vi "Timeout action.vi"(8 "error in (no error)":errorcluster, 11 "Loop data in":T1={"Config"={"List"=[], "max rows"=8, "Listbox placement"=enum."None", "String Color Options"={"Use? (F)"=FALSE, "Color - Valid"=0, "Color - Invalid"=0, "Allow blank?"=FALSE}}, "Refs"={"String"=refnum, "Listbox"=refnum}, "State"={"LB active?"=FALSE}}) -> (0 "error out":errorcluster, 3 "Loop data out":T1={"Config"={"List"=[], "max rows"=8, "Listbox placement"=enum."None", "String Color Options"={"Use? (F)"=FALSE, "Color - Valid"=0, "Color - Invalid"=0, "Allow blank?"=FALSE}}, "Refs"={"String"=refnum, "Listbox"=refnum}, "State"={"LB active?"=FALSE}})   [LabVIEW 2021, in "Autocomplete Textbox.lvlib"]
uses:
  Autocomplete Textbox.lvlib
  Loop Data.ctl
  Inputs.ctl
  Classes/Handle/Listbox placement.ctl
  Color String Options.ctl
  Refs.ctl
  State data.ctl
  Classes/Handle/Handle.lvclass
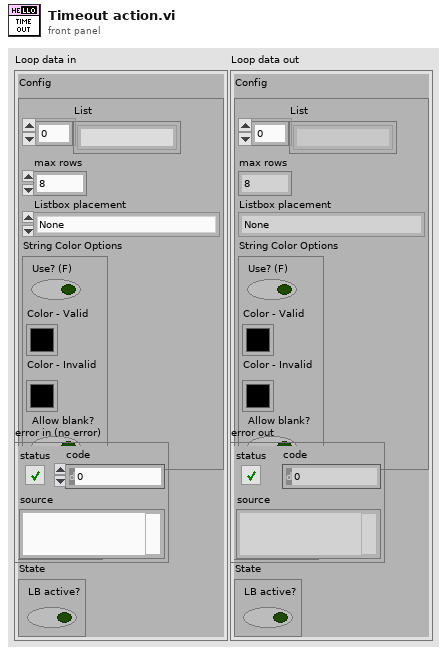
[diagram p1: front panel]
types:
  T1 = typedef "Autocomplete Textbox.lvlib/Loop Data.ctl" = cluster{"Config":T2, "Refs":T5, "State":T6}
  T2 = typedef "Autocomplete Textbox.lvlib/Inputs.ctl" = cluster{"List":string[], "max rows":i32, "Listbox placement":T3, "String Color Options":T4}
  T3 = typedef "Autocomplete Textbox.lvlib/Handle.lvclass/Listbox placement.ctl" = enum16{"None", "Under String", "Fit to Pane"}
  T4 = typedef "Autocomplete Textbox.lvlib/Color String Options.ctl" = cluster{"Use? (F)":bool, "Color - Valid":u32, "Color - Invalid":u32, "Allow blank?":bool}
  T5 = typedef "Autocomplete Textbox.lvlib/Refs.ctl" = cluster{"String":refnum<vi>, "Listbox":refnum<vi>}
  T6 = typedef "Autocomplete Textbox.lvlib/State data.ctl" = cluster{"LB active?":bool}
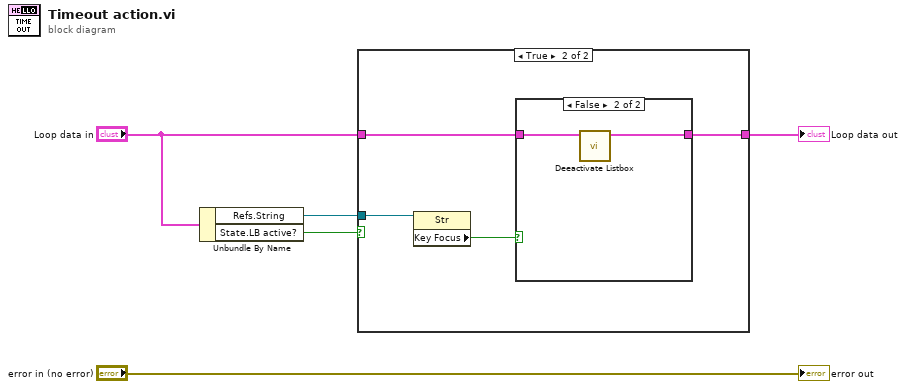
[diagram p0: block diagram]
diagram:
  n1 = Unbundle By Name("Loop data in") -> ("Refs.String"=w4:refnum<vi>, "State.LB active?"=w1:bool)
  n2 = case shown="True" w1 {
    tunnel: w4 -> [_ w10]
    tunnel: "Loop data in" -> [w6 w8]
    tunnel: [w6 w7] -> w2
    frame False {
    }
    frame True {
      n3 = property class="Str"(reference=w10) -> ("Key Focus"=w9:bool)  [unwired: 1 in, 2 out]
      n4 = case shown="False" w9 {
        tunnel: w8 -> [w11 w13]
        tunnel: [w11 w12] -> w7
        frame True {
        }
        frame False {
          n5 = call "Deeactivate Listbox.vi"("Loop data in"=w13) -> ("Loop data out"=w12:T1)  [unwired: 9 in, 1 out]
        }
      }
    }
  }
  "Loop data out" <- w2
  "error out" <- "error in (no error)"
